vi "Error Converter (ErrCode or Status).vi"(8 "error in (no error)":errorcluster, 10 "handle in":u64, 11 "error code":i32) -> (0 "error out":errorcluster)   [LabVIEW 2019, in "BTI429LV.lvlib"]
uses:
  Ballard - Arinc-429 Engine.llb/BTI429LV.lvlib
  Error Info.ctl
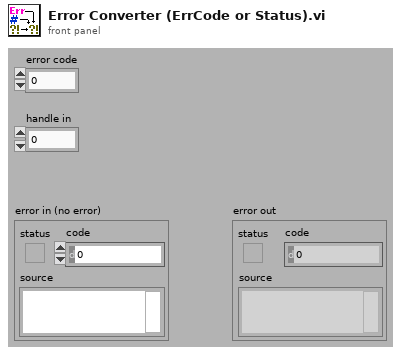
[diagram p1: front panel]
types:
  T1 = typedef "BTI429LV.lvlib/Error Info.ctl" = u32
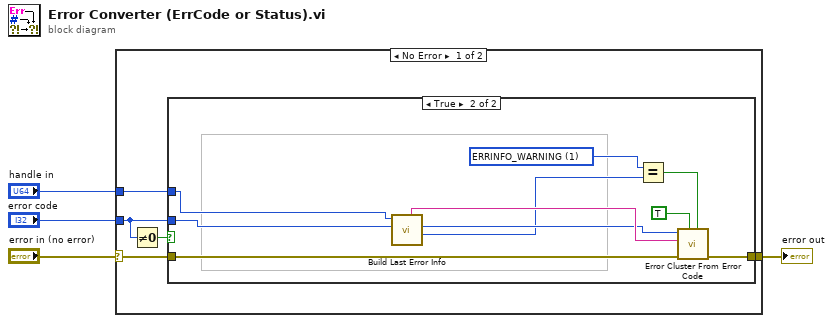
[diagram p0: block diagram]
diagram:
  n1 = case shown="No Error" "error in (no error)" {
    selector: "error in (no error)" -> [w8 w21]
    tunnel: [w6 w21] -> w3
    tunnel: "error code" -> [w7 _]
    tunnel: "handle in" -> [w5 _]
    frame No Error {
      n2 = Not Equal To 0?(x=w7) -> (x != 0?=w9:bool)
      n3 = case shown="True" w9 {
        tunnel: w8 -> [w10 w20]
        tunnel: w7 -> [_ w16]
        tunnel: [w10 w19] -> w6
        tunnel: w5 -> [_ w14]
        frame False {
        }
        frame True {
          w11 = T1 1 items=["ERRINFO_ERROR", "ERRINFO_WARNING", "ERRINFO_INFO"] ("error info")
          n4 = call "Build Last Error Info.vi"("error code in"=w16, "handle in"=w14) -> ("error info"=w13:T1, "error code out"=w15:i32, "error string out"=w17:string)  [unwired: 5 in, 2 out]
          n5 = Equal?(x=w11, y=w13) -> (x = y?=w12:bool)
          n6 = call "Error Cluster From Error Code.vi"("is warning? (False)"=w12, "show call chain? (False)"=TRUE, "error in (no error)"=w20, "error message (\"\")"=w17, "error code (0)"=w15) -> ("error out"=w19:errorcluster)  [unwired: 4 in]
        }
      }
    }
    frame Error {
    }
  }
  "error out" <- w3
